vi "Initialize Vivo Session.vi"(0 "resonator labels":string[](array[string]), 1 "Measurement Information In":T2={"Comments"="", "Directory Input"="", "Data file path"=path "C:/Data/EPR Data", "Scripting File"=path "C:/Data/Configuration Script.csv", "Save Data"=FALSE, "Tooth size (d11) [mm]"=0.0, "Tooth size (d12) [mm]"=0.0, "Tooth size (d21) [mm]"=0.0, "Tooth size (d22) [mm]"=0.0, "Dose of Tooth [Gy]"=0.0, "Safe Shutdown?"=FALSE, "Gases Available"=[], "Database Username"="", "Database Password"="", "Database Login URL"="", "Database Upload URL"="", "Database Success URL"="", "Database XML URL"="", "Database Resonator URL"="", "Session Number"=0, "Set #"=0, "Resonator Operator"="", "Session Type"="", "Tooth/Sample ID"="", "Volunteer ID"="", "Computer Operator"="", "Volunteer Type"="", "Site/Tooth Selection (T8,T9)"="", "Resonator"="", "Measurement Site"="", "Non-standard session?"=FALSE, "EPR DAQ Version"="", "Session Path"=path "C:/Data/EPR Data", "Chosen Applied State"="", "Chosen Initial State"="", "Time of Transition"="", "DAQ Mode"=enum."Engineering", "pO2/Scan [mmHg]"=[], "pO2/Set [mmHg]"=[], "Linewidth (HWHM)/Scan [Gauss]"=[], "Linewidth (HWHM)/Set [Gauss]"=[], "pO2 Conversion"="", "Dose Calibration Cluster"={"Dose Response"={"grand_mean"=0.0292016, "slope"=0.0188720543}, "Dose Correction"={"Sex"=1, "a0"=7.719669421, "a1"=-2.746550736, "a2"=-0.186490355, "a3"=0.041922063, "a4"=-0.849147359, "a5"=0.14330063, "a6"=0.019930219, "A_n"=40.0, "H_n"=10.12, "Dose Correction"=FALSE}, "Dose Reporting"={"Reporting is"=TRUE, "sd_threshold [AU]"=0.06, "sd_model [Gy]"=0.66, "dosimetric_threshold [Gy]"=2.0, "Add intrasession errors is"=FALSE, "Prior Radiation?"=FALSE}}, "OxyChip Slope"=0.0, "OxyChip Intercept"=0.0, "QA Mode"=enum."Select QA Mode", "QA Session?"=FALSE, "Sample Type"=enum."Empty Resonator", "Report pO2/Scan"=FALSE, "Skip End Session Save"=FALSE, "Number of sites"=enum."# Probes", "Recipient Name"="", "Sender Name"="", "Recipient Email"="", "Transition State History"=[], "pO2 Report Times"=[], "Temperature [C]"=0.0, "+Error pO2/Scan [mmHg]"=[], "-Error pO2/Scan [mmHg]"=[], "+Error pO2/Set [mmHg]"=[], "-Error pO2/Set [mmHg]"=[], "Oxy Phase Exclusion Tolerance [rad]"=0.0, "Oxy Center Exclusion Tolerance [%]"=0.0, "Oxy Exclude Unacceptable"=FALSE, "Oxy Unacceptable Estimate Flags"=[], "Save Session PPT"=FALSE, "Flagged Bad Sets"=[]} {"Oxy Center Exclusion Tolerance [%]" format="%#_9g"; "Oxy Phase Exclusion Tolerance [rad]" format="%#_9g"; "Temperature [C]" format="%#_9g"; "OxyChip Intercept" format="%#_9g"; "OxyChip Slope" format="%#_9g"; "Dose Calibration Cluster"."Dose Reporting"."dosimetric_threshold [Gy]" format="%#_9g"; "Dose Calibration Cluster"."Dose Reporting"."sd_model [Gy]" format="%#_9g"; "Dose Calibration Cluster"."Dose Reporting"."sd_threshold [AU]" format="%#_9g"; "Dose Calibration Cluster"."Dose Correction"."H_n" format="%#_9g"; "Dose Calibration Cluster"."Dose Correction"."A_n" format="%#_9g"; "Dose Calibration Cluster"."Dose Correction"."a6" format="%#.9g"; "Dose Calibration Cluster"."Dose Correction"."a5" format="%#.9g"; "Dose Calibration Cluster"."Dose Correction"."a4" format="%#.9g"; "Dose Calibration Cluster"."Dose Correction"."a3" format="%#.9g"; "Dose Calibration Cluster"."Dose Correction"."a2" format="%#.9g"; "Dose Calibration Cluster"."Dose Correction"."a1" format="%#.9g"; "Dose Calibration Cluster"."Dose Correction"."a0" format="%#.9g"; "Dose Calibration Cluster"."Dose Correction"."Sex" items=["Male"=1, "Female"=0]; "Dose Calibration Cluster"."Dose Response"."slope" format="%#_9g"; "Dose Calibration Cluster"."Dose Response"."grand_mean" format="%#_9g"}, 5 "Volunteer Selections":string[](array[string]), 9 "In Vivo Data File":string[](array[string])=["None v1", "T10-1 v1", "T10-10 v1", "T10-11 v1", "T10-12 v1", "T10-13 v1", "T10-14 v1", "T10-15 v1", "T10-16 v1", "T10-17 v1", "T10-2 v1", "T10-3 v1", "T10-4 v1", "T10-5 v1", "T10-6 v1", "T10-7 v1", "T10-8 v1", "T10-9 v1", "T1-10 v1", "T1-11 v1", "T11-1 v1", "T11-10 v1", "T11-11 v1", "T11-12 v1", "T11-13 v1", "T11-14 v1", "T11-15 v1", "T11-16 v1", "T11-17 v1", "T11-18 v1", "T11-19 v1", "T1-12 v1", "T11-2 v1", "T11-20 v1", "T11-21 v1", "T11-22 v1", "T11-23 v1", "T11-24 v1", "T11-25 v1", "T11-26 v1", "T11-27 v1", "T11-28 v1", "T11-29 v1", "T1-13 v1", "T11-3 v1", "T11-30 v1", "T11-31 v1", "T11-32 v1", "T11-33 v1", "T11-34 v1", "T11-35 v1", "T11-36 v1", "T11-37 v1", "T11-38 v1", "T11-39 v1", "T1-14 v1", "T11-4 v1", "T11-40 v1", "T11-41 v1", "T11-42 v1", "T1-15 v1", "T11-5 v1", "T1-16 v1", "T11-6 v1", "T1-17 v1", "T11-7 v1", "T1-18 v1", "T11-8 v1", "T1-19 v1", "T11-9 v1", "T1-2 v1", "T1-2 v2", "T1-2 v3", "T1-20 v1", "T1-21 v1", "T12-1 v1", "T12-10 v1", "T12-11 v1", "T12-12 v1", "T12-13 v1", "T12-14 v1", "T12-15 v1", "T12-16 v1", "T12-17 v1", "T12-18 v1", "T12-19 v1", "T1-22 v1", "T12-2 v1", "T1-23 v1", "T12-3 v1", "T1-24 v1", "T12-4 v1", "T1-25 v1", "T12-5 v1", "T1-26 v1", "T12-6 v1", "T1-27 v1", "T12-7 v1", "T1-28 v1", "T12-8 v1", "T1-29 v1", "T12-9 v1", "T1-3 v1", "T13-10 v1", "T13-11 v1", "T13-12 v1", "T13-13 v1", "T13-2 v1", "T13-3 v1", "T13-4 v1", "T13-5 v1", "T13-6 v1", "T13-7 v1", "T13-8 v1", "T13-9 v1", "T1-4 v1", "T14-1 v1", "T14-10 v1", "T14-11 v1", "T14-12 v1", "T14-13 v1", "T14-14 v1", "T14-15 v1", "T14-16 v1", "T14-17 v1", "T14-2 v1", "T14-3 v1", "T14-4 v1", "T14-5 v1", "T14-6 v1", "T14-7 v1", "T14-8 v1", "T14-9 v1", "T1-5 v1", "T1-5 v2", "T15-1 v1", "T15-10 v1", "T15-11 v1", "T15-2 v1", "T15-3 v1", "T15-4 v1", "T15-5 v1", "T15-6 v1", "T15-7 v1", "T15-8 v1", "T15-9 v1", "T1-6 v1", "T1-6 v2", "T16-1 v1", "T16-10 v1", "T16-11 v1", "T16-12 v1", "T16-13 v1", "T16-14 v1", "T16-15 v1", "T16-16 v1", "T16-17 v1", "T16-18 v1", "T16-19 v1", "T16-2 v1", "T16-20 v1", "T16-21 v1", "T16-22 v1", "T16-23 v1", "T16-24 v1", "T16-25 v1", "T16-3 v1", "T16-4 v1", "T16-5 v1", "T16-6 v1", "T16-7 v1", "T16-8 v1", "T16-9 v1", "T1-7 v1", "T17-1 v1", "T17-10 v1", "T17-11 v1", "T17-12 v1", "T17-13 v1", "T17-14 v1", "T17-15 v1", "T17-16 v1", "T17-17 v1", "T17-2 v1", "T17-3 v1", "T17-4 v1", "T17-5 v1", "T17-6 v1", "T17-7 v1", "T17-8 v1", "T17-9 v1", "T1-8 v1", "T18-1 v1", "T18-2 v1", "T18-3 v1", "T18-4 v1", "T18-5 v1", "T18-6 v1", "T18-7 v1", "T18-8 v1", "T18-9 v1", "T1-9 v1", "T19-1 v1", "T19-10 v1", "T19-11 v1", "T19-12 v1", "T19-13 v1", "T19-14 v1", "T19-15 v1", "T19-16 v1", "T19-17 v1", "T19-18 v1", "T19-19 v1", "T19-2 v1", "T19-3 v1", "T19-4 v1", "T19-5 v1", "T19-6 v1", "T19-7 v1", "T19-8 v1", "T19-9 v1", "T20-1 v1", "T20-10 v1", "T20-11 v1", "T20-12 v1", "T20-13 v1", "T20-14 v1", "T20-2 v1", "T20-3 v1", "T20-4 v1", "T20-5 v1", "T20-6 v1", "T20-7 v1", "T20-8 v1", "T20-9 v1", "T2-1 v1", "T2-10 v1", "T2-11 v1", "T21-1 v1", "T21-10 v1", "T21-11 v1", "T21-12 v1", "T21-13 v1", "T21-14 v1", "T21-15 v1", "T21-16 v1", "T21-17 v1", "T21-18 v1", "T21-19 v1", "T2-12 v1", "T21-20 v1", "T2-13 v1", "T21-3 v1", "T21-4 v1", "T21-5 v1", "T21-6 v1", "T21-7 v1", "T21-8 v1", "T21-9 v1", "T2-2 v1", "T22-1 v1", "T22-10 v1", "T22-11 v1", "T22-12 v1", "T22-13 v1", "T22-14 v1", "T22-15 v1", "T22-16 v1", "T22-17 v1", "T22-18 v1", "T22-19 v1", "T22-2 v1", "T22-3 v1", "T22-4 v1", "T22-5 v1", "T22-6 v1", "T22-7 v1", "T22-8 v1", "T22-9 v1", "T2-3 v1", "T23-1 v1", "T23-10 v1", "T23-11 v1", "T23-12 v1", "T23-13 v1", "T23-14 v1", "T23-15 v1", "T23-16 v1", "T23-17 v1", "T23-18 v1", "T23-19 v1", "T23-2 v1", "T23-20 v1", "T23-21 v1", "T23-22 v1", "T23-23 v1", "T23-24 v1", "T23-25 v1", "T23-3 v1", "T23-4 v1", "T23-5 v1", "T23-6 v1", "T23-7 v1", "T23-8 v1", "T23-9 v1", "T2-4 v1", "T24-1 v1", "T24-10 v1", "T24-11 v1", "T24-12 v1", "T24-13 v1", "T24-14 v1", "T24-2 v1", "T24-3 v1", "T24-4 v1", "T24-5 v1", "T24-6 v1", "T24-7 v1", "T24-8 v1", "T24-9 v1", "T2-5 v1", "T25-1 v1", "T25-10 v1", "T25-11 v1", "T25-12 v1", "T25-13 v1", "T25-14 v1", "T25-15 v1", "T25-16 v1", "T25-17 v1", "T25-18 v1", "T25-19 v1", "T25-2 v1", "T25-20 v1", "T25-21 v1", "T25-22 v1", "T25-23 v1", "T25-24 v1", "T25-25 v1", "T25-26 v1", "T25-27 v1", "T25-3 v1", "T25-4 v1", "T25-5 v1", "T25-6 v1", "T25-7 v1", "T25-8 v1", "T25-9 v1", "T2-6 v1", "T26-1 v1", "T26-10 v1", "T26-11 v1", "T26-12 v1", "T26-13 v1", "T26-14 v1", "T26-15 v1", "T26-16 v1", "T26-17 v1", "T26-18 v1", "T26-19 v1", "T26-2 v1", "T26-20 v1", "T26-21 v1", "T26-22 v1", "T26-23 v1", "T26-24 v1", "T26-25 v1", "T26-26 v1", "T26-3 v1", "T26-4 v1", "T26-5 v1", "T26-6 v1", "T26-7 v1", "T26-8 v1", "T26-9 v1", "T2-7 v1", "T27-1 v1", "T27-10 v1", "T27-11 v1", "T27-12 v1", "T27-13 v1", "T27-14 v1", "T27-15 v1", "T27-16 v1", "T27-17 v1", "T27-18 v1", "T27-19 v1", "T27-2 v1", "T27-20 v1", "T27-21 v1", "T27-22 v1", "T27-23 v1", "T27-24 v1", "T27-25 v1", "T27-3 v1", "T27-4 v1", "T27-5 v1", "T27-6 v1", "T27-7 v1", "T27-8 v1", "T27-9 v1", "T2-8 v1", "T28-1 v1", "T28-2 v1", "T28-3 v1", "T28-4 v1", "T28-5 v1", "T28-6 v1", "T28-7 v1", "T28-8 v1", "T2-9 v1", "T29-1 v1", "T29-10 v1", "T29-11 v1", "T29-12 v1", "T29-13 v1", "T29-14 v1", "T29-15 v1", "T29-16 v1", "T29-17 v1", "T29-18 v1", "T29-19 v1", "T29-2 v1", "T29-20 v1", "T29-3 v1", "T29-4 v1", "T29-5 v1", "T29-6 v1", "T29-7 v1", "T29-8 v1", "T29-9 v1", "T30-1 v1", "T30-10 v1", "T30-11 v1", "T30-12 v1", "T30-13 v1", "T30-14 v1", "T30-15 v1", "T30-16 v1", "T30-17 v1", "T30-18 v1", "T30-19 v1", "T30-2 v1", "T30-3 v1", "T30-4 v1", "T30-5 v1", "T30-6 v1", "T30-7 v1", "T30-8 v1", "T30-9 v1", "T3-1 v1", "T3-10 v1", "T3-11 v1", "T31-1 v1", "T3-12 v1", "T31-2 v1", "T3-13 v1", "T31-3 v1", "T3-14 v1", "T31-4 v1", "T3-15 v1", "T3-16 v1", "T3-2 v1", "T32-1 v1", "T32-10 v1", "T32-11 v1", "T32-12 v1", "T32-13 v1", "T32-14 v1", "T32-15 v1", "T32-16 v1", "T32-17 v1", "T32-18 v1", "T32-19 v1", "T32-2 v1", "T32-3 v1", "T32-4 v1", "T32-5 v1", "T32-6 v1", "T32-7 v1", "T32-8 v1", "T32-9 v1", "T3-3 v1", "T3-4 v1", "T3-5 v1", "T3-6 v1", "T3-7 v1", "T3-8 v1", "T3-9 v1", "T4-1 v1", "T4-10 v1", "T4-2 v1", "T4-3 v1", "T4-4 v1", "T4-5 v1", "T4-6 v1", "T4-7 v1", "T4-8 v1", "T4-9 v1", "T5-1 v1", "T5-10 v1", "T5-11 v1", "T5-12 v1", "T5-13 v1", "T5-14 v1", "T5-15 v1", "T5-16 v1", "T5-17 v1", "T5-18 v1", "T5-19 v1", "T5-2 v1", "T5-3 v1", "T5-4 v1", "T5-5 v1", "T5-6 v1", "T5-7 v1", "T5-8 v1", "T5-9 v1", "T6-1 v1", "T6-10 v1", "T6-11 v1", "T6-12 v1", "T6-13 v1", "T6-14 v1", "T6-15 v1", "T6-16 v1", "T6-17 v1", "T6-18 v1", "T6-19 v1", "T6-2 v1", "T6-20 v1", "T6-21 v1", "T6-22 v1", "T6-3 v1", "T6-4 v1", "T6-5 v1", "T6-6 v1", "T6-7 v1", "T6-8 v1", "T6-9 v1", "T7-1 v1", "T7-10 v1", "T7-11 v1", "T7-12 v1", "T7-13 v1", "T7-14 v1", "T7-15 v1", "T7-16 v1", "T7-17 v1", "T7-2 v1", "T7-3 v1", "T7-4 v1", "T7-5 v1", "T7-6 v1", "T7-7 v1", "T7-8 v1", "T7-9 v1", "T8-1 v1", "T8-10 v1", "T8-11 v1", "T8-12 v1", "T8-13 v1", "T8-14 v1", "T8-15 v1", "T8-16 v1", "T8-17 v1", "T8-18 v1", "T8-19 v1", "T8-2 v1", "T8-20 v1", "T8-21 v1", "T8-22 v1", "T8-23 v1", "T8-23 v2", "T8-24 v1", "T8-25 v1", "T8-26 v1", "T8-27 v1", "T8-28 v1", "T8-29 v1", "T8-3 v1", "T8-30 v1", "T8-31 v1", "T8-32 v1", "T8-33 v1", "T8-34 v1", "T8-35 v1", "T8-6 v1", "T8-7 v1", "T8-8 v1", "T8-9 v1", "T9-1 v1", "T9-10 v1", "T9-11 v1", "T9-12 v1", "T9-13 v1", "T9-14 v1", "T9-15 v1", "T9-16 v1", "T9-17 v1", "T9-18 v1", "T9-19 v1", "T9-2 v1", "T9-20 v1", "T9-21 v1", "T9-22 v1", "T9-23 v1", "T9-24 v1", "T9-3 v1", "T9-4 v1", "T9-5 v1", "T9-6 v1", "T9-7 v1", "T9-8 v1", "T9-9 v1", "V117-9 v1", "V125-9 v1"], 11 "Sample Selection":string[](array[string]), 12 "Tooth Position":string[](array[string])) -> (3 "Measurement Information Out":T2={"Comments"="", "Directory Input"="", "Data file path"=path "C:/Data/EPR Data", "Scripting File"=path "C:/Data/Configuration Script.csv", "Save Data"=FALSE, "Tooth size (d11) [mm]"=0.0, "Tooth size (d12) [mm]"=0.0, "Tooth size (d21) [mm]"=0.0, "Tooth size (d22) [mm]"=0.0, "Dose of Tooth [Gy]"=0.0, "Safe Shutdown?"=FALSE, "Gases Available"=[], "Database Username"="", "Database Password"="", "Database Login URL"="", "Database Upload URL"="", "Database Success URL"="", "Database XML URL"="", "Database Resonator URL"="", "Session Number"=0, "Set #"=0, "Resonator Operator"="", "Session Type"="", "Tooth/Sample ID"="", "Volunteer ID"="", "Computer Operator"="", "Volunteer Type"="", "Site/Tooth Selection (T8,T9)"="", "Resonator"="", "Measurement Site"="", "Non-standard session?"=FALSE, "EPR DAQ Version"="", "Session Path"=path "C:/Data/EPR Data", "Chosen Applied State"="", "Chosen Initial State"="", "Time of Transition"="", "DAQ Mode"=enum."Engineering", "pO2/Scan [mmHg]"=[], "pO2/Set [mmHg]"=[], "Linewidth (HWHM)/Scan [Gauss]"=[], "Linewidth (HWHM)/Set [Gauss]"=[], "pO2 Conversion"="", "Dose Calibration Cluster"={"Dose Response"={"grand_mean"=0.0292016, "slope"=0.0188720543}, "Dose Correction"={"Sex"=1, "a0"=7.719669421, "a1"=-2.746550736, "a2"=-0.186490355, "a3"=0.041922063, "a4"=-0.849147359, "a5"=0.14330063, "a6"=0.019930219, "A_n"=40.0, "H_n"=10.12, "Dose Correction"=FALSE}, "Dose Reporting"={"Reporting is"=TRUE, "sd_threshold [AU]"=0.06, "sd_model [Gy]"=0.66, "dosimetric_threshold [Gy]"=2.0, "Add intrasession errors is"=FALSE, "Prior Radiation?"=FALSE}}, "OxyChip Slope"=0.0, "OxyChip Intercept"=0.0, "QA Mode"=enum."Select QA Mode", "QA Session?"=FALSE, "Sample Type"=enum."Empty Resonator", "Report pO2/Scan"=FALSE, "Skip End Session Save"=FALSE, "Number of sites"=enum."# Probes", "Recipient Name"="", "Sender Name"="", "Recipient Email"="", "Transition State History"=[], "pO2 Report Times"=[], "Temperature [C]"=0.0, "+Error pO2/Scan [mmHg]"=[], "-Error pO2/Scan [mmHg]"=[], "+Error pO2/Set [mmHg]"=[], "-Error pO2/Set [mmHg]"=[], "Oxy Phase Exclusion Tolerance [rad]"=0.0, "Oxy Center Exclusion Tolerance [%]"=0.0, "Oxy Exclude Unacceptable"=FALSE, "Oxy Unacceptable Estimate Flags"=[], "Save Session PPT"=FALSE, "Flagged Bad Sets"=[]} {"Oxy Center Exclusion Tolerance [%]" format="%#_9g"; "Oxy Phase Exclusion Tolerance [rad]" format="%#_9g"; "Temperature [C]" format="%#_9g"; "OxyChip Intercept" format="%#_9g"; "OxyChip Slope" format="%#_9g"; "Dose Calibration Cluster"."Dose Reporting"."dosimetric_threshold [Gy]" format="%#_9g"; "Dose Calibration Cluster"."Dose Reporting"."sd_model [Gy]" format="%#_9g"; "Dose Calibration Cluster"."Dose Reporting"."sd_threshold [AU]" format="%#_9g"; "Dose Calibration Cluster"."Dose Correction"."H_n" format="%#_9g"; "Dose Calibration Cluster"."Dose Correction"."A_n" format="%#_9g"; "Dose Calibration Cluster"."Dose Correction"."a6" format="%#.9g"; "Dose Calibration Cluster"."Dose Correction"."a5" format="%#.9g"; "Dose Calibration Cluster"."Dose Correction"."a4" format="%#.9g"; "Dose Calibration Cluster"."Dose Correction"."a3" format="%#.9g"; "Dose Calibration Cluster"."Dose Correction"."a2" format="%#.9g"; "Dose Calibration Cluster"."Dose Correction"."a1" format="%#.9g"; "Dose Calibration Cluster"."Dose Correction"."a0" format="%#.9g"; "Dose Calibration Cluster"."Dose Correction"."Sex" items=["Male"=1, "Female"=0]; "Dose Calibration Cluster"."Dose Response"."slope" format="%#_9g"; "Dose Calibration Cluster"."Dose Response"."grand_mean" format="%#_9g"}, 4 "Sample Selection":string, 6 "Volunteer and Measurement ID":string="T10-10 v1", 8 "Sample Type":T1, 10 "Measurement Site":string, 14 "Selected Volunteer ID":string, 15 "Resonator ID":string="Inc2")   [LabVIEW 2016]
uses:
  Types/Measurement Information.ctl
  Analysis/Dose Calculation and Reporting/Dose Calculation Control.ctl
  Types/Sample Type.ctl
panel:
  in  "Tooth Height [mm]":dbl=10.12 format="%#_9g"
  in  "Age":dbl=40.0 format="%#_9g"
  in  "Sex":u16(ring)=1 items=["Male"=1, "Female"=0]
  in  "Subject reported prior irradiation?":bool
  in  "Measurement Site":i32(ring) items=["site1", "site2", "site3", "site4", "site5"]
  in  "Sample Selection":i32(ring) items=["LiPc", "OxyChip", "CarloErba", "Melanin", "Printex", "Char", "Other"]
  in  "Volunteer Type":i32(ring) items=["CarloErba", "Healthy", "Patient", "Animal", "OTHER"]
  in  "Volunteer ID":i32(ring) items=["V101", "V102", "V103", "V104", "V105", "V106", "V107", "V108", "V109", "V110", "Manual", ""]
  in  "Resonator":i32(ring) items=["", "3/1/2017 09:14:37 "]
  in  "Manual Entry":string
  in  "stop":bool
  # "EPR Input Parameters"
  # "Session Information"
  # "Oximetric Data and Information"
  # "Email"
  # "Tooth Information"
  # "Database"
  # "Session Information"
  # "Oximetric Data and Information"
  # "Email"
  # "Tooth Information"
  # "Database"
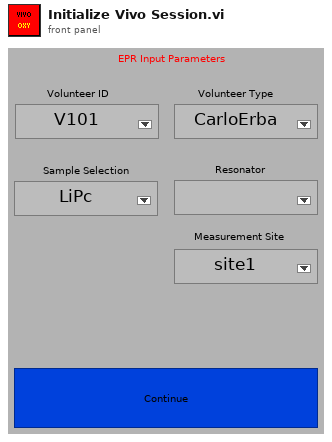
[diagram p1: front panel]
types:
  T1 = typedef "Sample Type.ctl" = enum16{"Empty Resonator", "IRS", "BallZero", "Irradiated Tooth", "Non-irradiated Tooth", "OxyChip", "LiPc", "PDT", "India Ink"}
  T2 = typedef "Measurement Information.ctl" = cluster{"Comments":string, "Directory Input":string, "Data file path":path, "Scripting File":path, "Save Data":bool, "Tooth size (d11) [mm]":dbl, "Tooth size (d12) [mm]":dbl, "Tooth size (d21) [mm]":dbl, "Tooth size (d22) [mm]":dbl, "Dose of Tooth [Gy]":dbl, "Safe Shutdown?":bool, "Gases Available":string[], "Database Username":string, "Database Password":string, "Database Login URL":string, "Database Upload URL":string, "Database Success URL":string, "Database XML URL":string, "Database Resonator URL":string, "Session Number":i32, "Set #":u32, "Resonator Operator":string, "Session Type":string, "Tooth/Sample ID":string, "Volunteer ID":string, "Computer Operator":string, "Volunteer Type":string, "Site/Tooth Selection (T8,T9)":string, "Resonator":string, "Measurement Site":string, "Non-standard session?":bool, "EPR DAQ Version":string, "Session Path":path, "Chosen Applied State":string, "Chosen Initial State":string, "Time of Transition":string, "DAQ Mode":enum16{"Engineering", "Dosimetry", "Oximetry"}, "pO2/Scan [mmHg]":dbl[][], "pO2/Set [mmHg]":dbl[][], "Linewidth (HWHM)/Scan [Gauss]":dbl[][], "Linewidth (HWHM)/Set [Gauss]":dbl[][], "pO2 Conversion":string, "Dose Calibration Cluster":T3, "OxyChip Slope":dbl, "OxyChip Intercept":dbl, "QA Mode":enum16{"Select QA Mode", "QA-Start/End", "QA-Mid", "QA-Weekly", "QA-Eng", "Check Calibration"}, "QA Session?":bool, "Sample Type":T1, "Report pO2/Scan":bool, "Skip End Session Save":bool, "Number of sites":enum16{"# Probes", "1", "2", "3", "4"}, "Recipient Name":string, "Sender Name":string, "Recipient Email":string, "Transition State History":string[], "pO2 Report Times":string[], "Temperature [C]":dbl, "+Error pO2/Scan [mmHg]":dbl[][], "-Error pO2/Scan [mmHg]":dbl[][], "+Error pO2/Set [mmHg]":dbl[][], "-Error pO2/Set [mmHg]":dbl[][], "Oxy Phase Exclusion Tolerance [rad]":dbl, "Oxy Center Exclusion Tolerance [%]":dbl, "Oxy Exclude Unacceptable":bool, "Oxy Unacceptable Estimate Flags":bool[], "Save Session PPT":bool, "Flagged Bad Sets":u32[]}
  T3 = typedef "Dose Calculation Control.ctl" = cluster{"Dose Response":cluster{"grand_mean":dbl, "slope":dbl}, "Dose Correction":cluster{"Sex":u16, "a0":dbl, "a1":dbl, "a2":dbl, "a3":dbl, "a4":dbl, "a5":dbl, "a6":dbl, "A_n":dbl, "H_n":dbl, "Dose Correction":bool}, "Dose Reporting":cluster{"Reporting is":bool, "sd_threshold [AU]":dbl, "sd_model [Gy]":dbl, "dosimetric_threshold [Gy]":dbl, "Add intrasession errors is":bool, "Prior Radiation?":bool}}
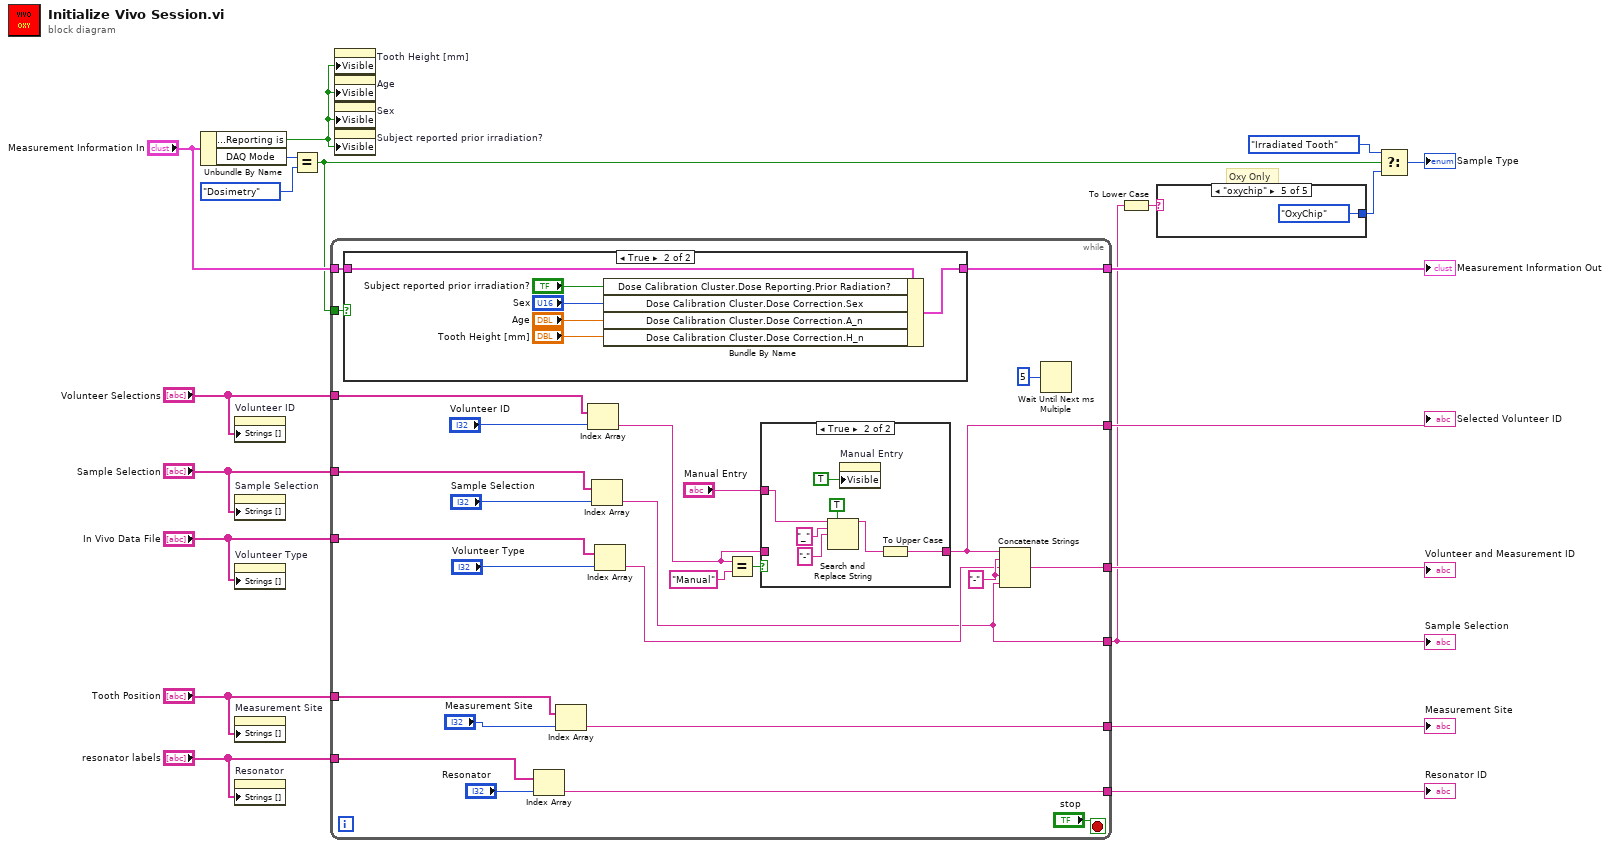
[diagram p0: block diagram]
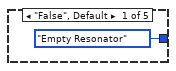
[diagram p2: hidden frame]
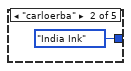
[diagram p3: hidden frame]
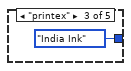
[diagram p4: hidden frame]
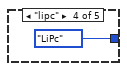
[diagram p5: hidden frame]
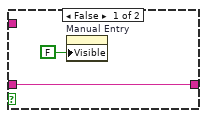
[diagram p7: hidden frame]
diagram:
  # "Oxy Only"
  n1 = Unbundle By Name("Measurement Information In") -> ("Dose Calibration Cluster.Dose Reporting.Reporting is"=w1:bool, "DAQ Mode"=w11:enum16{"Engineering", "Dosimetry", "Oximetry"})
  n2 = property on="Volunteer ID" class="Ring (strict)"("Strings []"="Volunteer Selections") -> ()  [unwired: 2 in, 2 out]
  n3 = property on="Sample Selection" class="Ring (strict)"("Strings []"="Sample Selection") -> ()  [unwired: 2 in, 2 out]
  n4 = property on="Volunteer Type" class="Ring (strict)"("Strings []"="In Vivo Data File") -> ()  [unwired: 2 in, 2 out]
  n5 = property on="Measurement Site" class="Ring (strict)"("Strings []"="Tooth Position") -> ()  [unwired: 2 in, 2 out]
  n6 = property on="Resonator" class="Ring (strict)"("Strings []"="resonator labels") -> ()  [unwired: 2 in, 2 out]
  n7 = Equal?(x=w11, y=enum16{"Engineering", "Dosimetry", "Oximetry"}."Dosimetry") -> (x = y?=w6:bool)
  n8 = while {
    tunnel: [w41] -> w20
    tunnel: "In Vivo Data File" -> [w37]
    tunnel: "Sample Selection" -> [w39]
    tunnel: "Volunteer Selections" -> [w38]
    tunnel: "resonator labels" -> [w36]
    tunnel: [w35] -> w18
    tunnel: "Tooth Position" -> [w29]
    tunnel: [w28] -> w14
    tunnel: [w26] -> w5
    tunnel: [w21] -> w12
    tunnel: "Measurement Information In" -> [w25]
    tunnel: w6 -> [w24]
    tunnel: [w23] -> w8
    stop <- "stop" stop-if-true
    w31 = "-" ("string")
    n9 = case shown="True" w24 {
      tunnel: w25 -> [w47 w53]
      tunnel: [w47 w52] -> w23
      frame False {
      }
      frame True {
        n10 = Bundle By Name(cluster=w53, "Dose Calibration Cluster.Dose Reporting.Prior Radiation?"="Subject reported prior irradiation?", "Dose Calibration Cluster.Dose Correction.Sex"="Sex", "Dose Calibration Cluster.Dose Correction.A_n"="Age", "Dose Calibration Cluster.Dose Correction.H_n"="Tooth Height [mm]") -> (w52:T2)
      }
    }
    n11 = Index Array(array=w36, index="Resonator") -> (element=w41:string)
    n12 = Index Array(array=w29, index="Measurement Site") -> (element=w28:string)
    n13 = Index Array(array=w38, index="Volunteer ID") -> (element=w22:string)
    n14 = Index Array(array=w39, index="Sample Selection") -> (element=w26:string)
    n15 = Index Array(array=w37, index="Volunteer Type") -> (element=w27:string)
    n16 = Equal?(x=w22, y="Manual") -> (x = y?=w44:bool)
    n17 = case shown="True" w44 {
      tunnel: w22 -> [w54 _]
      tunnel: "Manual Entry" -> [_ w57]
      tunnel: [w54 w61] -> w21
      frame False {
        n18 = property on="Manual Entry" class="Str"("Visible"=FALSE) -> ()  [unwired: 2 in, 2 out]
      }
      frame True {
        n19 = Search and Replace String(replace all?=TRUE ("replace all? (F)"), input string=w57, search string="_", replace string="-" ("replace string (\"\")")) -> (result string=w56:string)  [unwired: 4 in, 3 out]
        n20 = property on="Manual Entry" class="Str"("Visible"=TRUE) -> ()  [unwired: 2 in, 2 out]
        n21 = To Upper Case(1:w56) -> (0:w61:string)
      }
    }
    n22 = Concatenate Strings(w21, w31, w27, w31, w26) -> (w35:string)
    n23 = Wait Until Next ms Multiple(millisecond multiple=u32 5) -> ()  [unwired: 1 out]
  }
  "Volunteer and Measurement ID" <- w18
  "Resonator ID" <- w20
  "Measurement Site" <- w14
  "Sample Selection" <- w5
  "Selected Volunteer ID" <- w12
  "Measurement Information Out" <- w8
  n24 = property on="Tooth Height [mm]" class="DigNum (strict)"("Visible"=w1) -> ()  [unwired: 2 in, 2 out]
  n25 = property on="Age" class="DigNum (strict)"("Visible"=w1) -> ()  [unwired: 2 in, 2 out]
  n26 = property on="Sex" class="Ring (strict)"("Visible"=w1) -> ()  [unwired: 2 in, 2 out]
  n27 = property on="Subject reported prior irradiation?" class="Bool (strict)"("Visible"=w1) -> ()  [unwired: 2 in, 2 out]
  n28 = To Lower Case(string=w5) -> (all lower case string=w4:string)
  n29 = case shown="\"oxychip\"" w4 {
    tunnel: [Sample_Type."Empty Resonator" ("Sample Type") Sample_Type."India Ink" ("Sample Type") Sample_Type."India Ink" ("Sample Type") Sample_Type."LiPc" ("Sample Type") Sample_Type."OxyChip" ("Sample Type")] -> w3
    frame "False", Default {
    }
    frame "carloerba" {
    }
    frame "printex" {
    }
    frame "lipc" {
    }
    frame "oxychip" {
    }
  }
  n30 = Select(t=Sample_Type."Irradiated Tooth" ("Sample Type"), s=w6, f=w3) -> (s? t:f=→"Sample Type":T1)
